vi "LauncherAngle.vi"() -> ()   [LabVIEW 2012]
uses:
  State_Machine_Enum.ctl
  Robot Global Data.vi
  <vilib>/Rock Robotics/WPI/Relay/WPI_RelayValue.ctl
panel:
  in  "Start at bottom?":bool=TRUE
  in  "Use Encoder":bool
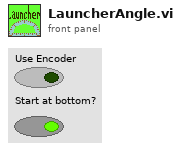
[diagram p1: front panel]
types:
  T1 = typedef "State_Machine_Enum.ctl" = enum16{"Idle", "Start", "Do", "Stop", "Init"}
  T2 = typedef "WPI_RelayValue.ctl" = enum16{"Off", "On", "Forward", "Reverse"}
  T3 = typedef "LoopDisable.ctl" = cluster{"Climb.vi":bool, "LauncherAngle.vi":bool, "Launcher.vi":bool, "ArmControl.vi":bool, "WinchMotor.vi":bool, "ReadDriveEncoder.vi":bool}
  T4 = typedef "WPI_DigitalInputDevRef.ctl" = cluster{"DevStatus":errorcluster, "DIO Channel":T5, "Digital Module":T6}
  T5 = typedef "FPGA_DIOChannel.ctl" = enum8{"DIO 1", "DIO 2", "DIO 3", "DIO 4", "DIO 5", "DIO 6", "DIO 7", "DIO 8", "DIO 9", "DIO 10", "DIO 11", "DIO 12", "DIO 13", "DIO 14", "Invalid"}
  T6 = typedef "FPGA_TypedefDigitalModule.ctl" = enum16{"Digital Module 1", "Digital Module 2"}
  T7 = typedef "WPI_EncoderDevRef.ctl" = cluster{"DevStatus":errorcluster, "EncoderIndex":T8, "CounterIndex":T9, "DistancePerCount":dbl, "Decoding Type":T10}
  T8 = typedef "FPGA_EncoderIdx.ctl" = enum8{"Enc 0", "Enc 1", "Enc 2", "Enc 3", "Invalid"}
  T9 = typedef "FPGA_CounterCtrSystemIndex.ctl" = enum8{"Ctr 0", "Ctr 1", "Ctr 2", "Ctr 3", "Ctr 4", "Ctr 5", "Ctr 6", "Ctr 7", "Invalid"}
  T10 = typedef "WPI_EncoderType.ctl" = enum16{"1x", "2x", "4x"}
  T11 = typedef "WPI_RelayDevRef.ctl" = cluster{"DevStatus":errorcluster, "Relay Channel":T12, "Digital Module":T6, "Relay Direction":T13}
  T12 = typedef "FPGA_DIORelayChannel.ctl" = enum8{"Relay 1", "Relay 2", "Relay 3", "Relay 4", "Relay 5", "Relay 6", "Relay 7", "Relay 8", "Invalid"}
  T13 = typedef "WPI_RelayDirection.ctl" = enum16{"Both directions", "Forward only", "Reverse only"}
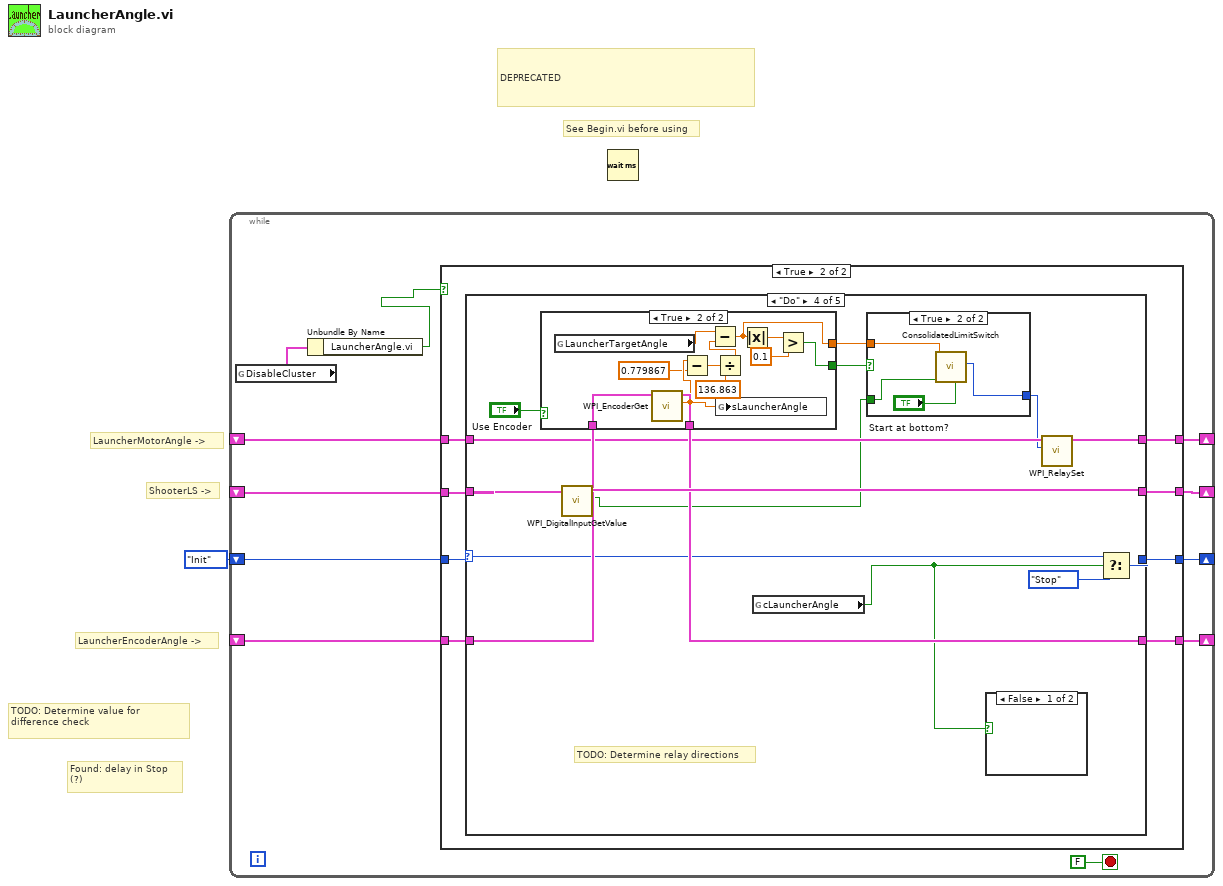
[diagram p0: block diagram]
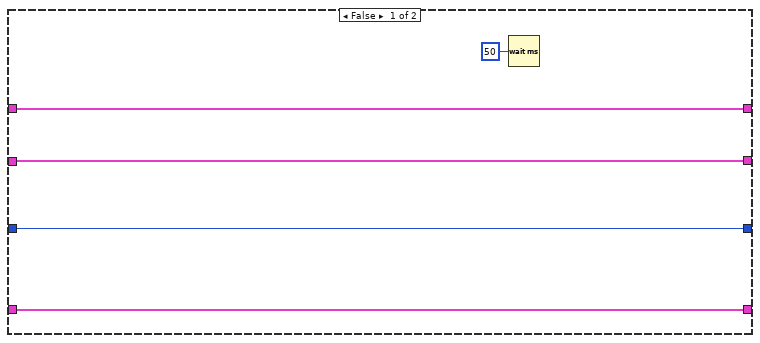
[diagram p2: hidden frame]
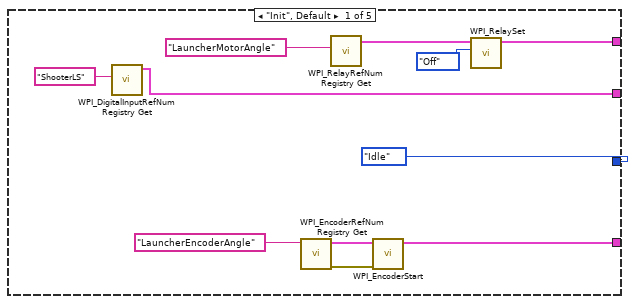
[diagram p3: hidden frame]
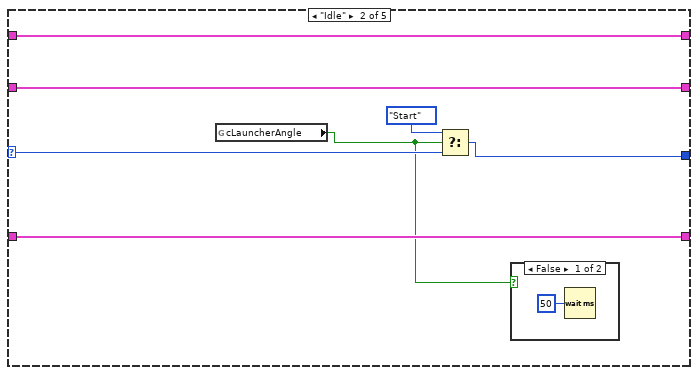
[diagram p4: hidden frame]
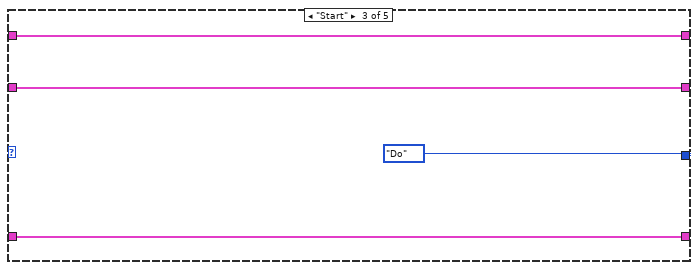
[diagram p6: hidden frame]
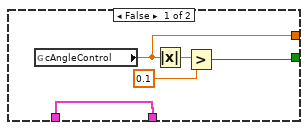
[diagram p7: hidden frame]
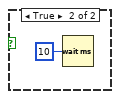
[diagram p8: hidden frame]
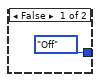
[diagram p9: hidden frame]
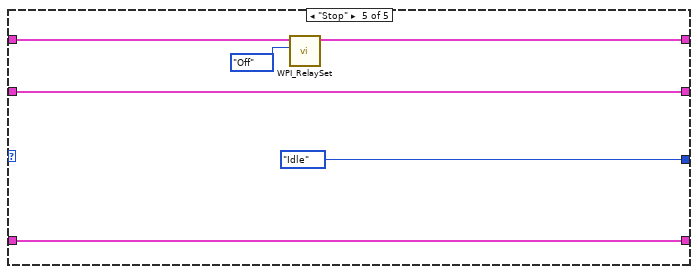
[diagram p10: hidden frame]
diagram:
  # "See Begin.vi before using"
  # "DEPRECATED"
  # "ShooterLS ->"
  # "Found: delay in Stop \n(?)"
  # "TODO: Determine value for difference check"
  # "LauncherEncoderAngle ->"
  # "LauncherMotorAngle ->"
  n1 = while {
    shift-right: [w10] -> _
    shift-left: State_Machine_Enum."Init" ("State") -> [w11]
    shift-right: [w9] -> _
    shift-left: _ -> [w8]
    shift-right: [w7] -> _
    shift-left: _ -> [w6]
    shift-right: [w4] -> _
    shift-left: _ -> [w5]
    stop <- FALSE stop-if-true
    n2 = global read "Robot Global Data.vi" "DisableCluster"() -> (w3:T3)
    n3 = Unbundle By Name(w3) -> ("LauncherAngle.vi"=w2:bool)
    n4 = case shown="True" w2 {
      tunnel: w11 -> [w15 w25]
      tunnel: [w15 w24] -> w10
      tunnel: [w14 w23] -> w9
      tunnel: w8 -> [w14 w22]
      tunnel: [w17 w21] -> w7
      tunnel: w6 -> [w17 w20]
      tunnel: w5 -> [w16 w19]
      tunnel: [w16 w18] -> w4
      frame False {
        n5 = Wait (ms)(milliseconds to wait=u32 50) -> ()  [unwired: 1 out]
      }
      frame True {
        n6 = case shown="\"Do\"" w25 {
          selector: w25 -> [_ w41 _ w58 _]
          tunnel: [State_Machine_Enum."Idle" ("State") w42 State_Machine_Enum."Do" ("State") w56 State_Machine_Enum."Idle" ("State")] -> w24
          tunnel: [w33 w38 w47 w59 w92] -> w23
          tunnel: w22 -> [_ w38 w47 w60 w92]
          tunnel: [w29 w40 w46 w57 w90] -> w21
          tunnel: w20 -> [_ w40 w46 w55 w91]
          tunnel: w19 -> [_ w39 w45 w63 w87]
          tunnel: [w26 w39 w45 w62 w87] -> w18
          frame "Init", Default {
            n7 = call <vilib>:"WPI_DigitalInputRefNum Registry Get.vi"("refnum name"="ShooterLS") -> ("DigitalInputDevRef"=w26:T4)  [unwired: 9 in, 1 out]
            n8 = call <vilib>:"WPI_EncoderRefNum Registry Get.vi"("refnum name"="LauncherEncoderAngle") -> ("error out"=w32:errorcluster, "EncoderDevRef"=w34:T7)  [unwired: 9 in]
            n9 = call <vilib>:"WPI_RelayRefNum Registry Get.vi"("refnum name"="LauncherMotorAngle") -> ("RelayDevRef"=w30:T11)  [unwired: 9 in, 1 out]
            n10 = call <vilib>:"WPI_EncoderStart.vi"("error in (no error)"=w32, "EncoderDevRef"=w34) -> ("EncoderDevRef"=w33:T7)  [unwired: 8 in, 1 out]
            n11 = call <vilib>:"WPI_RelaySet.vi"("RelayValue"=WPI_RelayValue."Off", "RelayDevRef"=w30) -> ("RelayDevRef"=w29:T11)  [unwired: 8 in, 1 out]
          }
          frame "Idle" {
            n12 = global read "Robot Global Data.vi" "cLauncherAngle"() -> (w37:bool)
            n13 = Select(t=State_Machine_Enum."Start" ("State"), s=w37, f=w41) -> (s? t:f=w42:T1)
            n14 = case shown="False" w37 {
              frame False {
                n15 = Wait (ms)(milliseconds to wait=u32 50) -> ()  [unwired: 1 out]
              }
              frame True {
              }
            }
          }
          frame "Start" {
          }
          frame "Do" {
            # "TODO: Determine relay directions"
            n16 = case shown="True" "Use Encoder" {
              tunnel: w60 -> [w64 w80]
              tunnel: [w64 w79] -> w59
              tunnel: [w65 w76] -> w54
              tunnel: [w66 w75] -> w51
              frame False {
                n17 = global read "Robot Global Data.vi" "cAngleControl"() -> (w65:dbl)
                n18 = Absolute Value(x=w65) -> (abs(x)=w68:dbl)
                n19 = Greater?(x=w68, y=0.1) -> (0:w66:bool)
              }
              frame True {
                n20 = global read "Robot Global Data.vi" "LauncherTargetAngle"() -> (w70:dbl)
                n21 = call <vilib>:"WPI_EncoderGet.vi"("EncoderDevRef"=w80) -> ("Distance"=w74:dbl, "EncoderDevRef"=w79:T7)  [unwired: 5 in, 4 out]
                n22 = Subtract(x=w74, y=0.779867) -> (x-y=w72:dbl)
                n23 = Divide(x=w72, y=136.863) -> (x/y=w69:dbl)
                n24 = Subtract(x=w70, y=w69) -> (x-y=w76:dbl)
                n25 = global write "Robot Global Data.vi" "sLauncherAngle"(w74) -> ()
                n26 = Absolute Value(x=w76) -> (abs(x)=w78:dbl)
                n27 = Greater?(x=w78, y=0.1) -> (0:w75:bool)
              }
            }
            n28 = call <vilib>:"WPI_DigitalInputGetValue.vi"("DigitalInputDevRef"=w63) -> ("Value"=w53:bool, "DigitalInputDevRef"=w62:T4)  [unwired: 8 in, 1 out]
            n29 = global read "Robot Global Data.vi" "cLauncherAngle"() -> (w49:bool)
            n30 = case shown="True" w51 {
              tunnel: w54 -> [_ w84]
              tunnel: w53 -> [_ w85]
              tunnel: [WPI_RelayValue."Off" ("RelayValue") w86] -> w52
              frame False {
              }
              frame True {
                n31 = call "ConsolidatedLimitSwitch.vi"("Start at bottom?"="Start at bottom?", "CurrentLSValue"=w85, "CurrentInput"=w84) -> ("RelayValue"=w86:T2)  [unwired: 8 in]
              }
            }
            n32 = case shown="False" w49 {
              frame False {
              }
              frame True {
                n33 = Wait (ms)(milliseconds to wait=u32 10) -> ()  [unwired: 1 out]
              }
            }
            n34 = call <vilib>:"WPI_RelaySet.vi"("RelayValue"=w52, "RelayDevRef"=w55) -> ("RelayDevRef"=w57:T11)  [unwired: 8 in, 1 out]
            n35 = Select(t=w58, s=w49, f=State_Machine_Enum."Stop" ("State")) -> (s? t:f=w56:T1)
          }
          frame "Stop" {
            n36 = call <vilib>:"WPI_RelaySet.vi"("RelayValue"=WPI_RelayValue."Off", "RelayDevRef"=w91) -> ("RelayDevRef"=w90:T11)  [unwired: 8 in, 1 out]
          }
        }
      }
    }
  }
  n37 = Wait (ms)() -> ()  [unwired: 1 in, 1 out]
